vi "PIDantiWindup.vi"(8 "PID Gains":cluster{"Kp":dbl, "Kd":dbl, "Ki":dbl}, 9 "Saturation":dbl, 10 "Position":dbl, 11 "Reference":dbl) -> (3 "control":dbl)   [LabVIEW 2018, in "kevLib2011.lvlib"]
uses:
  kevLib2011.lvlib
panel:
  # "Not Tested Yet"
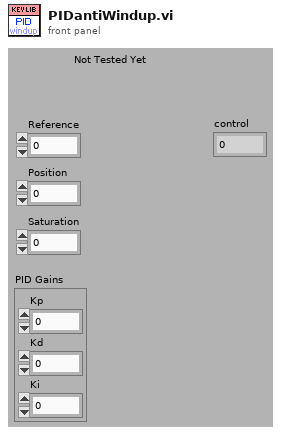
[diagram p1: front panel]
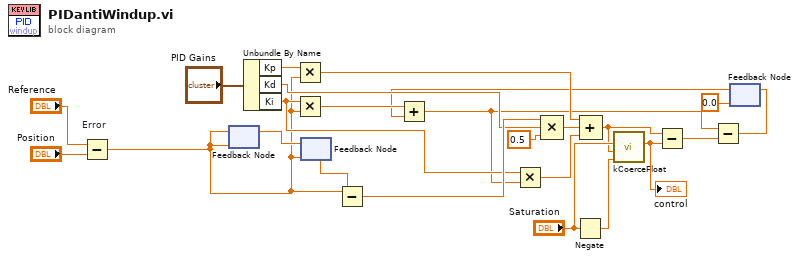
[diagram p0: block diagram]
diagram:
  n1 = Subtract "Error"(x="Reference", y="Position") -> (x-y=w10:dbl)
  n2 = feedback-in #1(w10) -> ()
  n3 = feedback #1(w10) -> (w19:dbl)
  n4 = Unbundle By Name("PID Gains") -> ("Kp"=w21:dbl, "Kd"=w16:dbl, "Ki"=w11:dbl)
  n5 = Multiply(x=w21, y=w10) -> (x*y=w20:dbl)
  n6 = Multiply(x=w11, y=w10) -> (x*y=w9:dbl)
  n7 = feedback-in #2(w19) -> ()
  n8 = feedback #2(w10) -> (w18:dbl)
  n9 = Subtract(x=w10, y=w18) -> (x-y=w17:dbl)
  n10 = Compound Arithmetic op=MULTIPLY(w17, w16, 0.5 ("value")) -> (w14:dbl)
  n11 = Negate(x="Saturation") -> (-x=w6:dbl)
  n12 = feedback #3(0.0 ("value")) -> (w8:dbl)
  n13 = Add(x=w9, y=w8) -> (x+y=w2:dbl)
  n14 = Multiply(x=w11, y=w2) -> (x*y=w12:dbl)
  n15 = Compound Arithmetic op=ADD(w20, w14, w12) -> (w5:dbl)
  n16 = call "kCoerceFloat.vi"("lower"=w6, "input"=w5, "upper"="Saturation") -> ("output"=w4:dbl)  [unwired: 7 in, 1 out]
  "control" <- w4
  n17 = Subtract(x=w5, y=w4) -> (x-y=w3:dbl)
  n18 = Subtract(x=w2, y=w3) -> (x-y=w1:dbl)
  n19 = feedback-in #3(w1) -> ()
